vi "ConfigWFG.vi"(0 "object in":refnum<class "AD2_SDK.lvclass">, 2 "Config(var)":variant, 5 "error in (no error)":errorcluster) -> (14 "object out":refnum<class "AD2_SDK.lvclass">, 19 "error out":errorcluster)   [LabVIEW 2021, in "AD2_SDK.lvclass"]
uses:
  AD2_SDK.lvclass
  AD2_WFG_SDK_class/WFG.ctl
  AD2_WFG_SDK_class/WFGCh.ctl
  AD2_WFG_SDK_class/AD2TriggerSources.ctl
  AD2_SDK.lvclass/AD2_SDK.ctl
  AD2_WFG_SDK_class/AD2_WFG_SDK.lvclass
panel:
  in  "WFGConfig":T1={"Running"=FALSE, "Ch1"={"idxChannel"=0, "Settings out of range"=FALSE, "Carrier"={"Frequency (Hz)"=0.0, "Amplitude (V)"=1.0, "Offset(V)"=0.0, "Symmetry(%) "=50.0, "Phase(Deg)"=0.0, "Function"=0, "Enable"=FALSE}, "Trigger"={"secRun(0=Cont)"=0.0, "secWait"=0.0, "cRepeat(0=inf)"=0, "Repeat Trigger"=FALSE, "TrigrSrc"=enum."trigrsrcNone"}, "FM Mod"={"Frequency (Hz)"=1000.0, "Amplitude (%)"=1.0, "Offset(V)"=0.0, "Symmetry(%) "=50.0, "Phase(Deg)"=0.0, "Function 2"=1, "Enable"=FALSE}}, "Ch2"={"idxChannel"=1, "Settings out of range"=FALSE, "Carrier"={"Frequency (Hz)"=1000.0, "Amplitude (V)"=1.0, "Offset(V)"=0.0, "Symmetry(%) "=50.0, "Phase(Deg)"=0.0, "Function"=1, "Enable"=FALSE}, "Trigger"={"secRun(0=Cont)"=0.0, "secWait"=0.0, "cRepeat(0=inf)"=0, "Repeat Trigger"=FALSE, "TrigrSrc"=enum."trigrsrcNone"}, "FM Mod"={"Frequency (Hz)"=1000.0, "Amplitude (%)"=1.0, "Offset(V)"=0.0, "Symmetry(%) "=50.0, "Phase(Deg)"=0.0, "Function 2"=1, "Enable"=FALSE}}, "SyncronizeState"=enum."Independent"} {"Ch2"."FM Mod"."Function 2" items=["DC"=0, "Sine"=1, "Square"=2, "Triangle"=3, "RampUp"=4, "RampDown"=5, "Noise"=6, "Pulse"=7, "Custom"=30]; "Ch2"."Carrier"."Function" items=["DC"=0, "Sine"=1, "Square"=2, "Triangle"=3, "RampUp"=4, "RampDown"=5, "Noise"=6, "Pulse"=7, "Custom"=30]; "Ch1"."FM Mod"."Function 2" items=["DC"=0, "Sine"=1, "Square"=2, "Triangle"=3, "RampUp"=4, "RampDown"=5, "Noise"=6, "Pulse"=7, "Custom"=30]; "Ch1"."Carrier"."Function" items=["DC"=0, "Sine"=1, "Square"=2, "Triangle"=3, "RampUp"=4, "RampDown"=5, "Noise"=6, "Pulse"=7, "Custom"=30]}
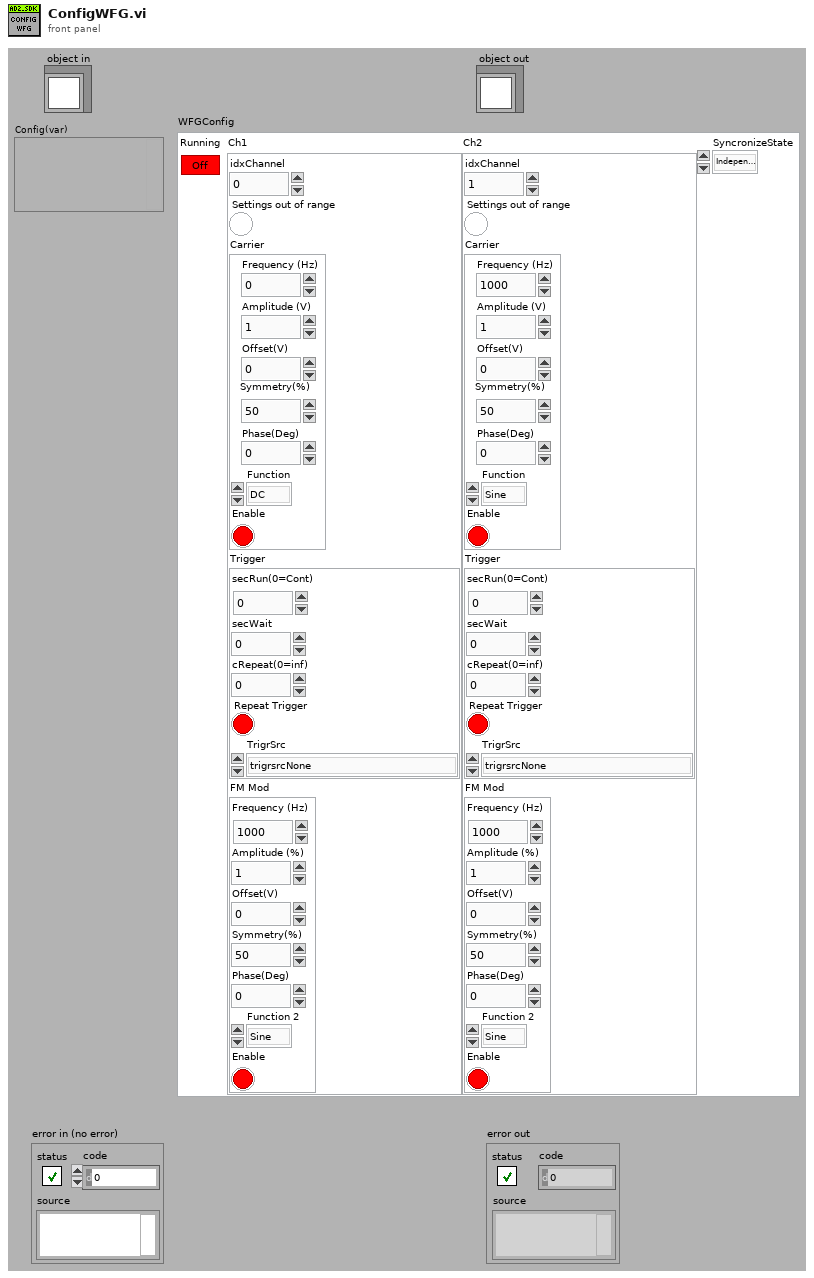
[diagram p1: front panel]
types:
  T1 = typedef "AD2_WFG_SDK.lvclass/WFG.ctl" = cluster{"Running":bool, "Ch1":T2, "Ch2":T2, "SyncronizeState":enum16{"Independent", "Ch1Master", "Ch2Master"}}
  T2 = typedef "AD2_WFG_SDK.lvclass/WFGCh.ctl" = cluster{"idxChannel":i32, "Settings out of range":bool, "Carrier":cluster{"Frequency (Hz)":dbl, "Amplitude (V)":dbl, "Offset(V)":dbl, "Symmetry(%) ":dbl, "Phase(Deg)":dbl, "Function":u16, "Enable":bool}, "Trigger":cluster{"secRun(0=Cont)":dbl, "secWait":dbl, "cRepeat(0=inf)":i32, "Repeat Trigger":bool, "TrigrSrc":T3}, "FM Mod":cluster{"Frequency (Hz)":dbl, "Amplitude (%)":dbl, "Offset(V)":dbl, "Symmetry(%) ":dbl, "Phase(Deg)":dbl, "Function 2":u16, "Enable":bool}}
  T3 = typedef "AD2_SDK.lvclass/AD2TriggerSources.ctl" = enum8{"trigrsrcNone", "trigsrcPC", "trigsrcDetectorAnalogIn", "trigsrcDetectorDigitalIn", "trigsrcAnalogIn", "trigsrcDigitalIn", "trigsrcDigitalOut", "trigsrcAnalogOut1", "trigsrcAnalogOut2", "trigsrcAnalogOut3", "trigsrcAnalogOut4", "trigsrcExternal1", "trigsrcExternal2", "trigsrcExternal3", "trigsrcExternal4", ""}
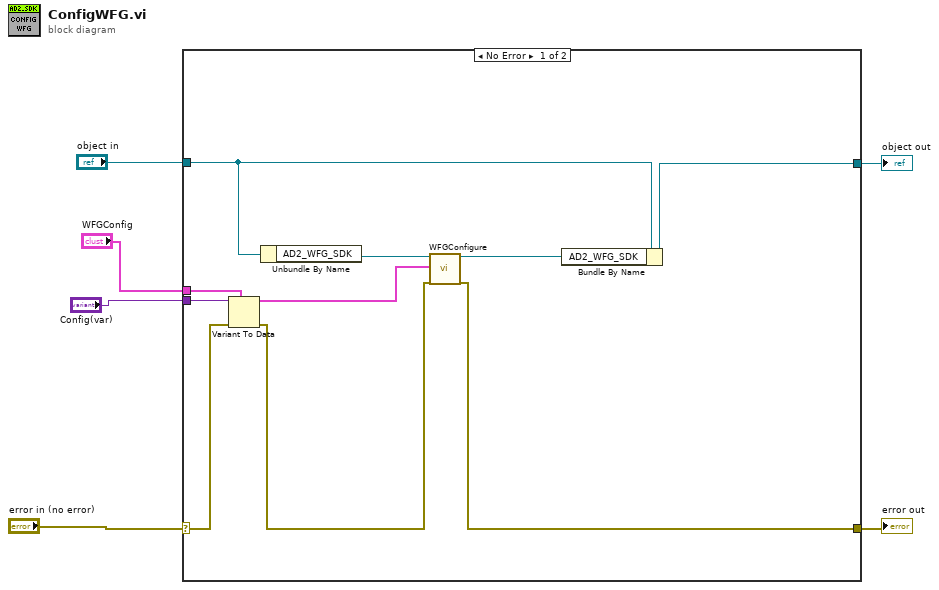
[diagram p0: block diagram]
diagram:
  n1 = case shown="No Error" "error in (no error)" {
    selector: "error in (no error)" -> [w8 w18]
    tunnel: [w12 w18] -> w5
    tunnel: [w15 w17] -> w3
    tunnel: "object in" -> [w16 w17]
    tunnel: "Config(var)" -> [w11 _]
    tunnel: "WFGConfig" -> [w10 _]
    frame No Error {
      n2 = Variant To Data(error in=w8, type=w10, Variant=w11) -> (data=w9:T1, error out=w7:errorcluster)
      n3 = Unbundle By Name(w16) -> ("AD2_WFG_SDK"=w14:refnum<class "AD2_WFG_SDK.lvclass">)
      n4 = call-dynamic "WFGConfigure.vi"("object in"=w14, "WFGConfig"=w9, "error in (no error)"=w7) -> ("object out"=w13:refnum<class "AD2_WFG_SDK.lvclass">, "error out"=w12:errorcluster)  [unwired: 14 in, 1 out]
      n5 = Bundle By Name(cluster=w16, "AD2_WFG_SDK"=w13) -> (w15:refnum<class "AD2_SDK.lvclass">)
    }
    frame Error {
    }
  }
  "error out" <- w5
  "object out" <- w3
